vi "cleanup_vi.vi"(11 "vi id":string) -> (0 "error out":errorcluster)   [LabVIEW 2020]
doc: "Cleans up the block diagram of a vi referenced by reference number. Use this at the end of a new VI creation to make sure everything looks nice and clean."
uses:
  G-AI Core/G-AI Core.lvlib
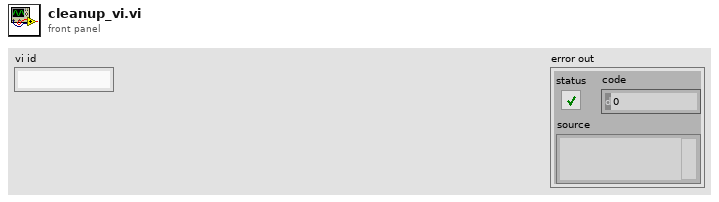
[diagram p1: front panel]
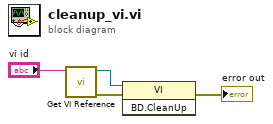
[diagram p0: block diagram]
diagram:
  n1 = call "Get VI Reference.vi"("id"="vi id") -> ("error out"=w1:errorcluster, "vi reference"=w2:refnum<vi>)  [unwired: 9 in]
  n2 = invoke class="VI" method="BD.CleanUp"(reference=w2, error in=w1) -> (error out=→"error out":errorcluster)  [unwired: 1 in, 2 out]
